vi "Trial 7.vi"() -> ()   [LabVIEW 2022 SP3]
panel:
  out "Detect car entry":bool[](array[boolean])
  out "Parking slot announcement":string
  out "Parking slot left":dbl
  out "Availability":string
  in  "start":bool
  out "Vehicle Count":dbl
  in  "stop":bool
  out "Parking Zone 1, 2, 3\nAvailability (Full)":bool[](array[boolean])
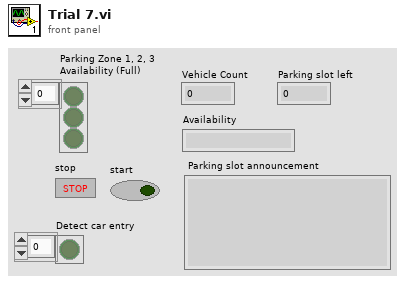
[diagram p1: front panel]
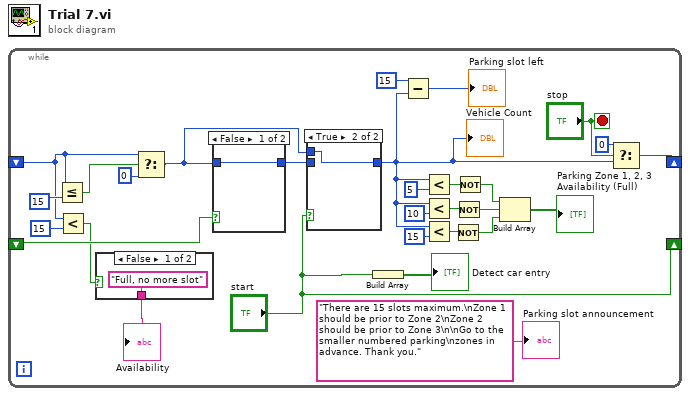
[diagram p0: block diagram]
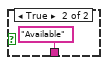
[diagram p2: hidden frame]
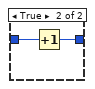
[diagram p4: hidden frame]
diagram:
  n1 = while {
    shift-right: [w14] -> _
    shift-left: _ -> [w18]
    shift-right: ["start"] -> _
    shift-left: _ -> [w27]
    stop <- "stop" stop-if-true
    n2 = Less Or Equal?(x=w18, y=15) -> (x <= y?=w21:bool)
    n3 = Less?(x=w18, y=15) -> (x < y?=w16:bool)
    n4 = case shown="False" w16 {
      tunnel: ["Full, no more slot" "Available"] -> w24
      frame False {
      }
      frame True {
      }
    }
    "Availability" <- w24
    n5 = Select(t=w18, s=w21, f=0) -> (s? t:f=w22:i32)
    n6 = case shown="False" w27 {
      tunnel: w22 -> [w34 w36]
      tunnel: [w34 w35] -> w28
      frame False {
      }
      frame True {
        n7 = Increment(x=w36) -> (x+1=w35:i32)
      }
    }
    n8 = case shown="True" "start" {
      tunnel: w28 -> [w32 _]
      tunnel: [w32 w33] -> w11
      tunnel: w22 -> [_ w33]
      frame False {
      }
      frame True {
      }
    }
    "Vehicle Count" <- w11
    n9 = Build Array("start") -> (→"Detect car entry":bool[])
    n10 = Subtract(x=15, y=w11) -> (x-y=→"Parking slot left":i32)
    n11 = Less?(x=w11, y=5) -> (x < y?=w8:bool)
    n12 = Less?(x=w11, y=10) -> (x < y?=w7:bool)
    n13 = Less?(x=w11, y=15) -> (x < y?=w6:bool)
    n14 = Not(x=w6) -> (.not. x?=w3:bool)
    n15 = Not(x=w7) -> (.not. x?=w4:bool)
    n16 = Not(x=w8) -> (.not. x?=w5:bool)
    n17 = Build Array(w5, w4, w3) -> (→"Parking Zone 1, 2, 3\nAvailability (Full)":bool[])
    n18 = Select(t=0, s="stop", f=w11) -> (s? t:f=w14:i32)
    "Parking slot announcement" <- "There are 15 slots maximum.\nZone 1 should be prior to Zone 2\nZone 2 should be prior to Zone 3\n\nGo to the smaller numbered parking\nzones in advance. Thank you."
  }
